vi "Sort Color Map.vi"(11 "colorMap":string) -> (3 "Parsed Color Map":T1[](array[typedef]))   [LabVIEW 2019, in "LSS.lvlib"]
doc: "Parse a colorMap string input into it's corresponding LSS properties.\n\n<b>Inputs:</b>\n<b>colorMap</b> - This string is an LSS formatted string that allows the mapping of hexidecimal color constants to string names that are easier to remember. Once a color is defined in the colorMap, any subsequent LSS call can simply use the name of the color instead of the hexidecimal representation. This input is only used when the mode input is set to \"Write\" or \"Add\". The format for this string is as follows:\n colorMap{\n myColorName:#000000;\n}\n\n<b>Outputs:</b>\n<b>Parsed colorMap</b> - Contains the colorMap information parsed into an array that can be used to map color mnemonics to hexidecimal representations."
uses:
  LSS.lvlib
  Controls/colorMap.ctl
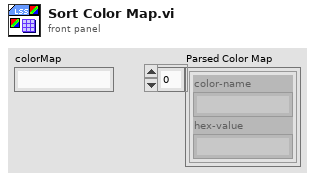
[diagram p1: front panel]
types:
  T1 = typedef "LSS.lvlib/colorMap.ctl" = cluster{"color-name":string, "hex-value":string}
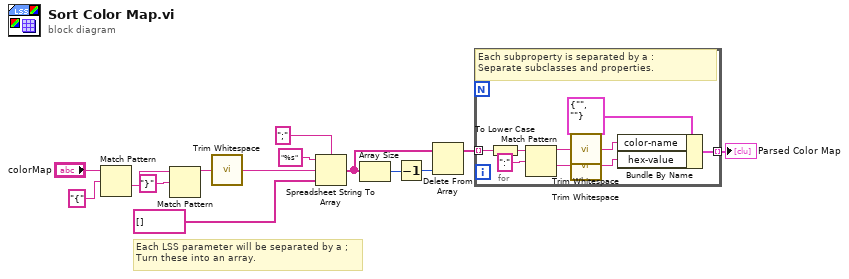
[diagram p0: block diagram]
diagram:
  # "Each LSS parameter will be separated by a ;\nTurn these into an array."
  n1 = Match Pattern(string="colorMap", regular expression="{" ("search string/char (-)")) -> (after substring=w4:string)  [unwired: 1 in, 3 out]
  n2 = Match Pattern(string=w4, regular expression="}" ("search string/char (-)")) -> (before substring=w11:string)  [unwired: 1 in, 3 out]
  n3 = call <vilib>:"Trim Whitespace.vi"("string"=w11) -> ("trimmed string"=w8:string)  [unwired: 1 in]
  n4 = Spreadsheet String To Array(delimiter (Tab)=";", format string="%s", spreadsheet string=w8, array type (2D Dbl)=string[] [] ("appended array")) -> (array=w5:string[])
  n5 = Array Size(array=w5) -> (size(s)=w6:i32)
  n6 = Decrement(x=w6) -> (x-1=w12:i32)
  n7 = Delete From Array(array=w5, index=w12) -> (array with subset deleted=w13:string[])  [unwired: 1 in, 1 out]
  n8 = for {
    tunnel: w13 -> [w23] mode=indexing
    tunnel: [w22] -> w14 mode=indexing
    # "Each subproperty is separated by a :\nSeparate subclasses and properties."
    n9 = To Lower Case(string=w23) -> (all lower case string=w15:string)
    n10 = Match Pattern(string=w15, regular expression=":") -> (before substring=w21:string, after substring=w20:string)  [unwired: 1 in, 2 out]
    n11 = call <vilib>:"Trim Whitespace.vi"("string"=w21) -> ("trimmed string"=w17:string)  [unwired: 1 in]
    n12 = call <vilib>:"Trim Whitespace.vi"("string"=w20) -> ("trimmed string"=w16:string)  [unwired: 1 in]
    n13 = Bundle By Name(cluster=T1 {"color-name"="", "hex-value"=""}, "color-name"=w17, "hex-value"=w16) -> (w22:T1)
  }
  "Parsed Color Map" <- w14
